vi "DataSocket Read Connections Manager.vi"(7 "Action":enum16{"Get", "Close", "Close All"}(ring), 11 "URL":string) -> (3 "connection id":refnum<k13>)   [LabVIEW 2023, in "Reply Msg DataSocket.lvclass"]
uses:
  Reply Msg DataSocket.lvclass
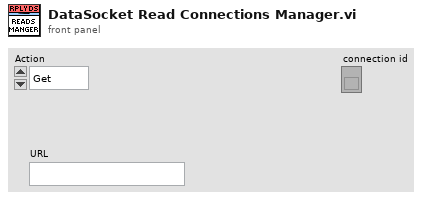
[diagram p1: front panel]
types:
  T1 = enum16{"Read", "Write", "ReadWrite", "BufferedRead", "BufferedReadWrite"}
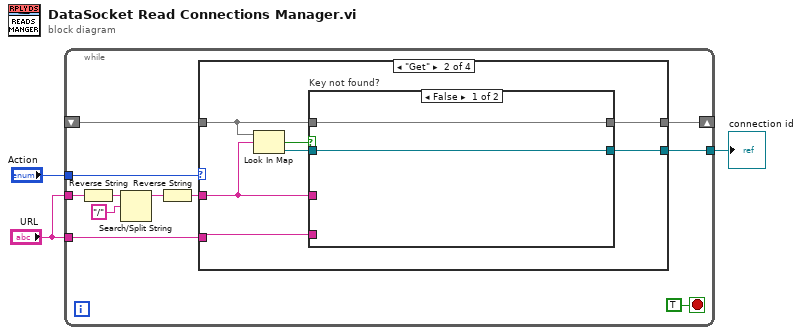
[diagram p0: block diagram]
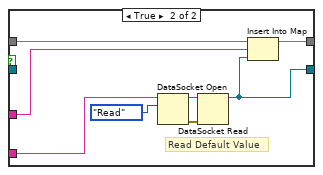
[diagram p3: hidden frame]
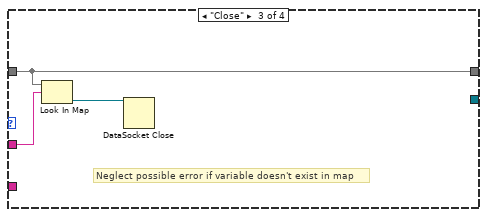
[diagram p4: hidden frame]
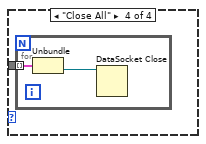
[diagram p5: hidden frame]
diagram:
  n1 = while {
    shift-right: [w12] -> _
    shift-left: _ -> [w11]
    tunnel: "URL" -> [w6]
    tunnel: [w10] -> w2
    tunnel: "Action" -> [w13]
    tunnel: "URL" -> [w4]
    stop <- TRUE stop-if-true
    n2 = Reverse String(1:w6) -> (0:w9:string)
    n3 = Search/Split String(string=w9, search string/char (-)="/") -> (substring before match=w7:string)  [unwired: 1 in, 2 out]
    n4 = Reverse String(1:w7) -> (0:w5:string)
    n5 = case shown="\"Get\"" w13 {
      tunnel: [_ w19 w32 _] -> w12
      tunnel: w11 -> [_ w20 w32 w35]
      tunnel: w5 -> [_ w18 w34 _]
      tunnel: [_ w16 _ _] -> w10
      tunnel: w4 -> [_ w15 _ _]
      frame Default {
      }
      frame "Get" {
        n6 = Look In Map(map=w20, key=w18) -> (key not found?=w21:bool, value=w17:refnum<k13>)  [unwired: 1 in]
        n7 = case "Key not found?" shown="False" w21 {
          tunnel: w20 -> [w22 w31]
          tunnel: [w22 w30] -> w19
          tunnel: w18 -> [_ w24]
          tunnel: w17 -> [w23 _]
          tunnel: [w23 w27] -> w16
          tunnel: w15 -> [_ w25]
          frame False {
          }
          frame True {
            # "Read Default Value"
            n8 = DataSocket Open(10:T1."Read" ("mode"), 11:w25) -> (0:w26:errorcluster, 3:w28:refnum<k13>)  [unwired: 2 in]
            n9 = DataSocket Read(8:w26, 11:w28) -> (3:w27:refnum<k13>)  [unwired: 3 in, 6 out]
            n10 = Insert Into Map(map in=w31, key=w24, value=w27) -> (map out=w30:map{string, refnum<k13>})  [unwired: 2 out]
          }
        }
      }
      frame "Close" {
        # "Neglect possible error if variable doesn't exist in map"
        n11 = Look In Map(map=w32, key=w34) -> (value=w33:refnum<k13>)  [unwired: 1 in, 1 out]
        n12 = DataSocket Close(11:w33) -> ()  [unwired: 2 in, 2 out]
      }
      frame "Close All" {
        n13 = for {
          tunnel: w35 -> [w37] mode=indexing
          n14 = Unbundle(w37) -> ("connection id"=w36:refnum<k13>)  [unwired: 1 out]
          n15 = DataSocket Close(11:w36) -> ()  [unwired: 2 in, 2 out]
        }
      }
    }
  }
  "connection id" <- w2
